vi "Tset正弦波生成.vi"() -> ()   [LabVIEW 2019]
panel:
  out "波形图表":dbl[](graph)
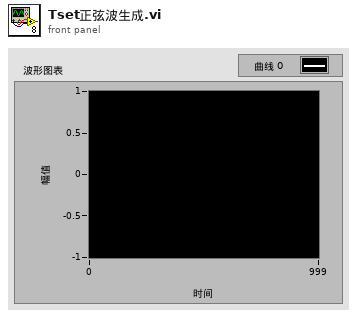
[diagram p1: front panel]
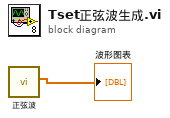
[diagram p0: block diagram]
diagram:
  n1 = call "正弦波.vi"() -> ("Sine 波形"=→"波形图表":dbl[])  [unwired: 10 in, 1 out]
